vi "init.vi"(8 "error in (no error)":errorcluster, 11 "A in":refnum<class "A.lvclass">) -> (0 "error out":errorcluster, 3 "A out":refnum<class "A.lvclass">)   [LabVIEW 2015, in "A.lvclass"]
uses:
  A.lvclass
  General.lvclass
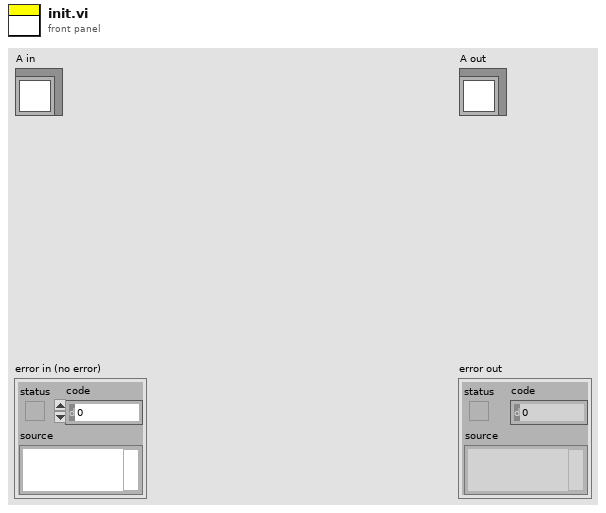
[diagram p1: front panel]
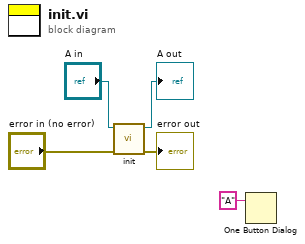
[diagram p0: block diagram]
diagram:
  n1 = call-parent "init.vi"("error in (no error)"="error in (no error)", "General in"="A in") -> ("error out"=→"error out":errorcluster, "General out"=→"A out":refnum<class "A.lvclass">)  [unwired: 8 in]
  n2 = One Button Dialog(message="A") -> ()  [unwired: 1 in, 1 out]
